vi "MPU char to digital data.vi"(8 "Error In":errorcluster, 10 "MPU characteristic data":u8[](array[numeric])) -> (0 "Error Out":errorcluster, 2 "Digital MPU data":T1)   [LabVIEW 2016]
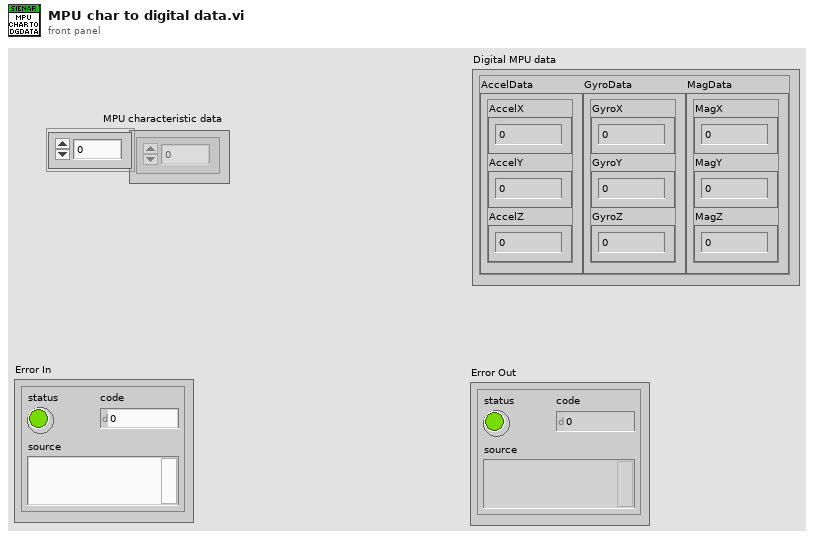
[diagram p1: front panel]
types:
  T1 = cluster{"AccelData":cluster{"AccelX":i16, "AccelY":i16, "AccelZ":i16}, "GyroData":cluster{"GyroX":i16, "GyroY":i16, "GyroZ":i16}, "MagData":cluster{"MagX":i16, "MagY":i16, "MagZ":i16}}
  T2 = cluster{cluster{"[0]":i16, "[1]":i16, "[2]":i16}, cluster{"[0]":i16, "[1]":i16, "[2]":i16}, cluster{"[0]":i16, "[1]":i16, "[2]":i16}}
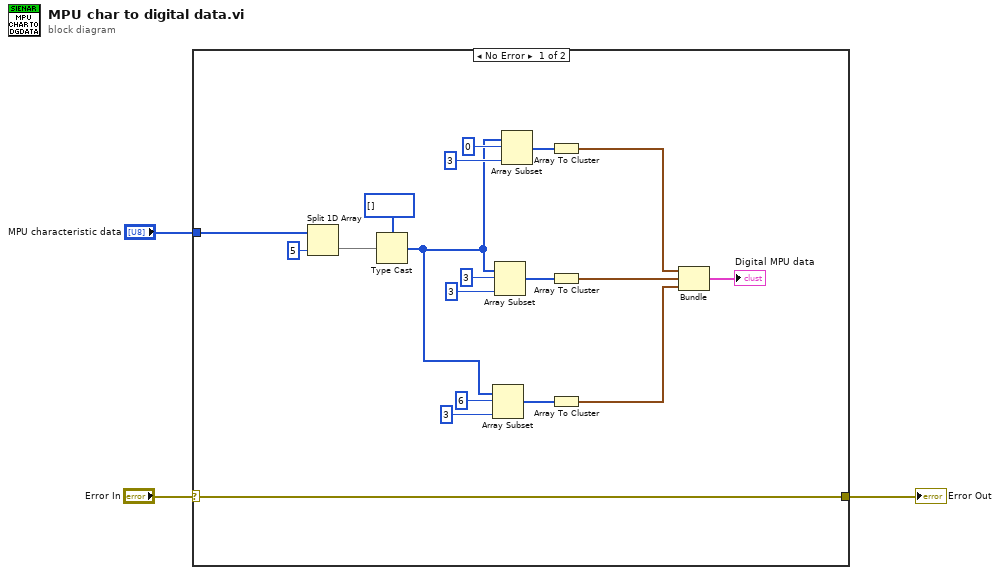
[diagram p0: block diagram]
diagram:
  n1 = case shown="No Error" "Error In" {
    selector: "Error In" -> [w14 w23]
    tunnel: "MPU characteristic data" -> [w15 _]
    tunnel: [w14 w23] -> w1
    frame No Error {
      n2 = Split 1D Array(array=w15, index=5) -> (second subarray=w21:u8[])  [unwired: 1 out]
      n3 = Type Cast(type=i16[] [], x=w21) -> (*(type *) &x=w11:i16[])
      n4 = Array Subset(array=w11, index=6, length=3) -> (w8:i16[])
      n5 = Array Subset(array=w11, index=3, length=3) -> (w9:i16[])
      n6 = Array Subset(array=w11, index=0, length=3) -> (w10:i16[])
      n7 = Array To Cluster(array=w10) -> (cluster=w7:cluster{"[0]":i16, "[1]":i16, "[2]":i16})
      n8 = Array To Cluster(array=w9) -> (cluster=w6:cluster{"[0]":i16, "[1]":i16, "[2]":i16})
      n9 = Array To Cluster(array=w8) -> (cluster=w5:cluster{"[0]":i16, "[1]":i16, "[2]":i16})
      n10 = Bundle(w7, w6, w5) -> (→"Digital MPU data":T2)  [unwired: 1 in]
    }
    frame Error {
    }
  }
  "Error Out" <- w1
